vi "LoadMatrixData_Delay.vi"(8 "Nd":i16, 11 "NS":i16) -> (2 "done":bool)   [LabVIEW 2017]
uses:
  <vilib>/rvi/interface/RandomDataEmulation/niFpgaRandomDataHandleErrors.vi
  <vilib>/rvi/DataTransferAndStorage/Container/Common/niFpgaContainerExecOnDevCompGetState.vi
  <vilib>/rvi/Emulation/niFpgaEmulationIsFPGAContextNoSignature.vi
  <vilib>/rvi/DataTransferAndStorage/Container/Common/niFpgaContainerGetUniqueNameForEmu.vi
  <vilib>/rvi/Emulation/niFpgaProcessEmulError.vi
  <vilib>/rvi/Emulation/niFpgaSctlEmulationGetInTimedLoop.vi
  <vilib>/rvi/errors/nirviReportUnexpectedCaseInternalError (U32).vi
  <vilib>/rvi/Memory/Memory_Emulation/niFpgaMemoryEmulationCacheClearOnFirstRun.vi
  <vilib>/rvi/Memory/Memory_Emulation/nirvimemoryEmulationManagerCache_MakeExclusive.vi
  <vilib>/rvi/Memory/Memory_Emulation/niFpgaMemoryEmulationValidateCache.vi
  <vilib>/rvi/Memory/Memory_Emulation/nirvimemoryEmulationManagerCache_InsertValue.vi
  <vilib>/Utility/error.llb/Clear Errors.vi
  <vilib>/rvi/Memory/Memory_Emulation/nirvimemoryEmulationManagerCache_ReleaseExclusive.vi
  <vilib>/rvi/Memory/Memory_Emulation/nirvimemoryEmulationManagerCache_GetValue.vi
  <vilib>/rvi/Memory/Memory_Emulation/nirvimemoryEmulationManagerCache_SetValue.vi
  <vilib>/rvi/Emulation/niFpgaSctlEmulationResourceMgr.vi
  <vilib>/rvi/DataTransferAndStorage/Container/XNode/niFpgaContainer.xnode
  <vilib>/rvi/interface/RandomDataEmulation/nirviRandomDataFpgaReadWriteTemplate.vi
  <vilib>/rvi/Memory/Memory_Emulation/niFpgaMemoryEmulationRefIn.vi
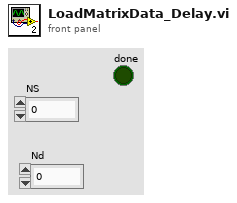
[diagram p1: front panel]
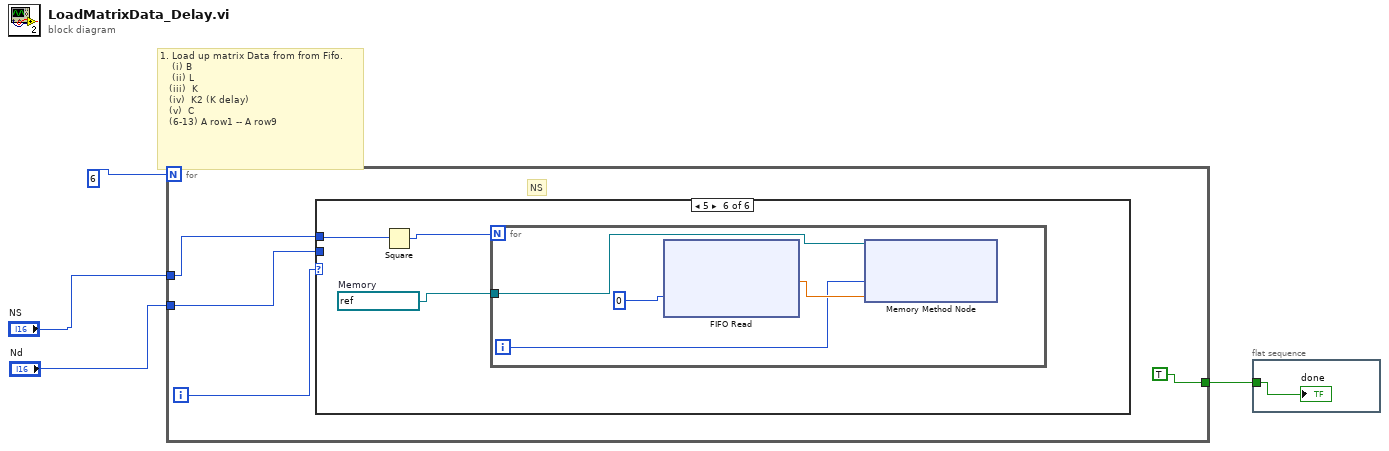
[diagram p0: block diagram]
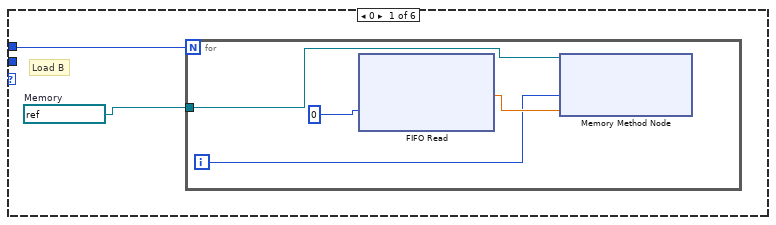
[diagram p2: hidden frame]
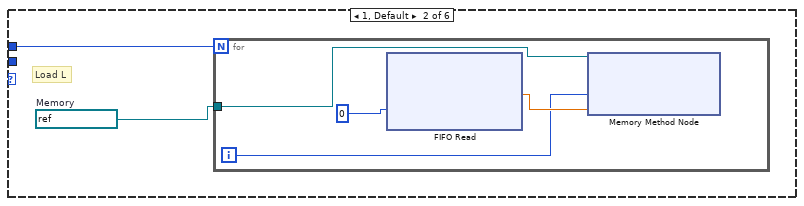
[diagram p3: hidden frame]
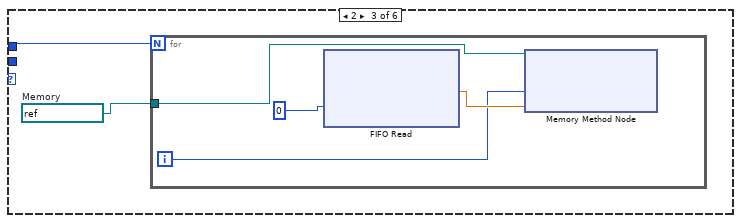
[diagram p4: hidden frame]
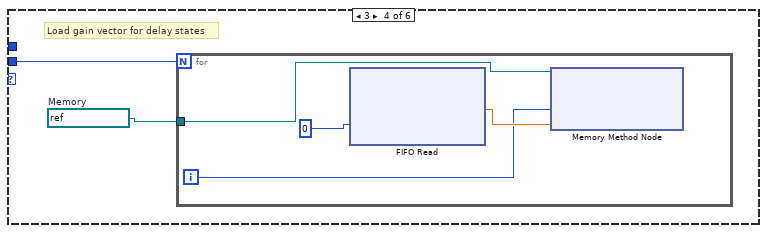
[diagram p5: hidden frame]
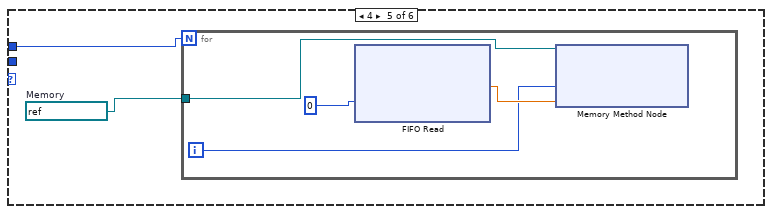
[diagram p6: hidden frame]
diagram:
  # "1. Load up matrix Data from from Fifo.\n    (i) B\n    (ii) L\n   (iii)  K\n   (iv)  K2 (K delay)\n   (v)  C\n   (6-13) A row1 -- A row9"
  n1 = for {
    N: i16 6 -> [_]
    tunnel: "NS" -> [w7]
    tunnel: [TRUE] -> w3
    tunnel: "Nd" -> [w5]
    i -> [w8]
    # "NS"
    n2 = case shown="5" w8 {
      tunnel: w7 -> [w9 w15 w21 _ w33 w39]
      tunnel: w5 -> [_ _ _ w27 _ _]
      frame 0 {
        w10 = refnum<k21> "Bz"  # Memory
        # "Load B"
        n3 = for {
          N: w9 -> [_]
          tunnel: w10 -> [w12]
          i -> [w11]
          n4 = xnode ("FIFO Read")("Timeout"=i16 0) -> ("Element"=w14:sgl)  [unwired: 1 in, 2 out]
          n5 = xnode ("Memory Method Node")("Address"=w11, "Data"=w14, "Memory In"=w12) -> ()  [unwired: 1 out]
        }
      }
      frame 1, Default {
        w16 = refnum<k21> "L"  # Memory
        # "Load L"
        n6 = for {
          N: w15 -> [_]
          tunnel: w16 -> [w18]
          i -> [w17]
          n7 = xnode ("FIFO Read")("Timeout"=i16 0) -> ("Element"=w20:sgl)  [unwired: 1 in, 2 out]
          n8 = xnode ("Memory Method Node")("Address"=w17, "Data"=w20, "Memory In"=w18) -> ()  [unwired: 1 out]
        }
      }
      frame 2 {
        w22 = refnum<k21> "K"  # Memory
        n9 = for {
          N: w21 -> [_]
          tunnel: w22 -> [w24]
          i -> [w23]
          n10 = xnode ("FIFO Read")("Timeout"=i16 0) -> ("Element"=w26:sgl)  [unwired: 1 in, 2 out]
          n11 = xnode ("Memory Method Node")("Address"=w23, "Data"=w26, "Memory In"=w24) -> ()  [unwired: 1 out]
        }
      }
      frame 3 {
        w28 = refnum<k21> "K2"  # Memory
        # "Load gain vector for delay states"
        n12 = for {
          N: w27 -> [_]
          tunnel: w28 -> [w30]
          i -> [w29]
          n13 = xnode ("FIFO Read")("Timeout"=i16 0) -> ("Element"=w32:sgl)  [unwired: 1 in, 2 out]
          n14 = xnode ("Memory Method Node")("Address"=w29, "Data"=w32, "Memory In"=w30) -> ()  [unwired: 1 out]
        }
      }
      frame 4 {
        w34 = refnum<k21> "C"  # Memory
        n15 = for {
          N: w33 -> [_]
          tunnel: w34 -> [w36]
          i -> [w35]
          n16 = xnode ("FIFO Read")("Timeout"=i16 0) -> ("Element"=w38:sgl)  [unwired: 1 in, 2 out]
          n17 = xnode ("Memory Method Node")("Address"=w35, "Data"=w38, "Memory In"=w36) -> ()  [unwired: 1 out]
        }
      }
      frame 5 {
        w41 = refnum<k21> "AasCol"  # Memory
        n18 = Square(x=w39) -> (x^2=w40:i16)
        n19 = for {
          N: w40 -> [_]
          tunnel: w41 -> [w43]
          i -> [w42]
          n20 = xnode ("FIFO Read")("Timeout"=i16 0) -> ("Element"=w45:sgl)  [unwired: 1 in, 2 out]
          n21 = xnode ("Memory Method Node")("Address"=w42, "Data"=w45, "Memory In"=w43) -> ()  [unwired: 1 out]
        }
      }
    }
  }
  n22 = flat-sequence {
    tunnel: w3 -> [w46]
    frame #0 {
      "done" <- w46
    }
  }
